vi "TEST_ProgressLib.vi"() -> ()   [LabVIEW 2021]
uses:
  builds/ProgressLib/Progress.lvlibp/Progress.lvclass
panel:
  out "error out":errorcluster
  in  "Nb Element":u64=40
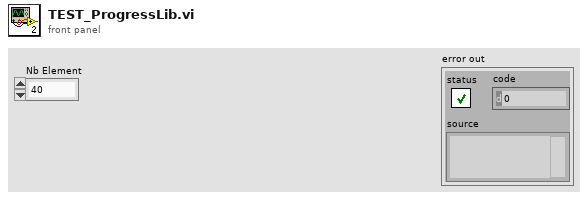
[diagram p1: front panel]
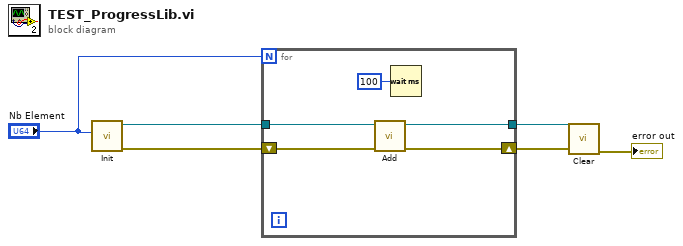
[diagram p0: block diagram]
diagram:
  n1 = call "Init.vi"("Nb Element"="Nb Element") -> ("error out"=w6:errorcluster, "Progress out"=w1:refnum<class "Progress.lvclass">)  [unwired: 9 in]
  n2 = for {
    N: "Nb Element" -> [_]
    tunnel: w1 -> [w11]
    tunnel: [w8] -> w4
    shift-right: [w7] -> w3
    shift-left: w6 -> [w10]
    n3 = call "Add.vi"("error in (no error)"=w10, "Progress in"=w11) -> ("error out"=w7:errorcluster, "Progress out"=w8:refnum<class "Progress.lvclass">)  [unwired: 8 in]
    n4 = Wait (ms)(milliseconds to wait=u32 100) -> ()  [unwired: 1 out]
  }
  n5 = call "Clear.vi"("error in (no error)"=w3, "Progress in"=w4) -> ("error out"=→"error out":errorcluster)  [unwired: 9 in]
